vi "Configure Marker.vi"(0 "VISA resource name":refnum<visa-resource-name>, 1 "Marker X Units (0: Seconds)":i32(ring) items=["Seconds", "Hertz"], 2 "Marker Y Position (0.0)":dbl, 5 "Marker Name (1: Marker 1)":i32(ring)=1 items=["Marker 1"=1, "Marker 2"=2], 7 "Marker Type (0: Off)":i32(ring) items=["Off", "Measurement", "Manual", "Waveform", "Binary", "Hex"], 9 "Marker X Position (0.0)":dbl, 11 "error in (no error)":errorcluster, 12 "Marker Source (0: Channel 1)":i32(ring) items=["Channel 1", "Channel 2", "Channel 3", "Channel 4", "Math", "Waveform Memory 1", "Waveform Memory 2"], 13 "Marker Y Units (0: Volts)":i32(ring) items=["Volts", "dB"]) -> (4 "VISA resource name out":refnum<visa-resource-name>, 15 "error out":errorcluster)   [LabVIEW 2010, in "Agilent 2000 3000 X-Series.lvlib"]
doc: "Configures the marker settings."
uses:
  <instrlib>/Agilent 2000 3000 X-Series/Agilent 2000 3000 X-Series.lvlib
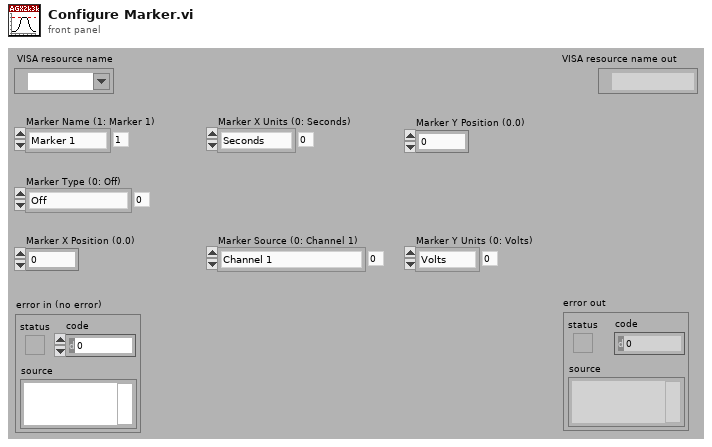
[diagram p1: front panel]
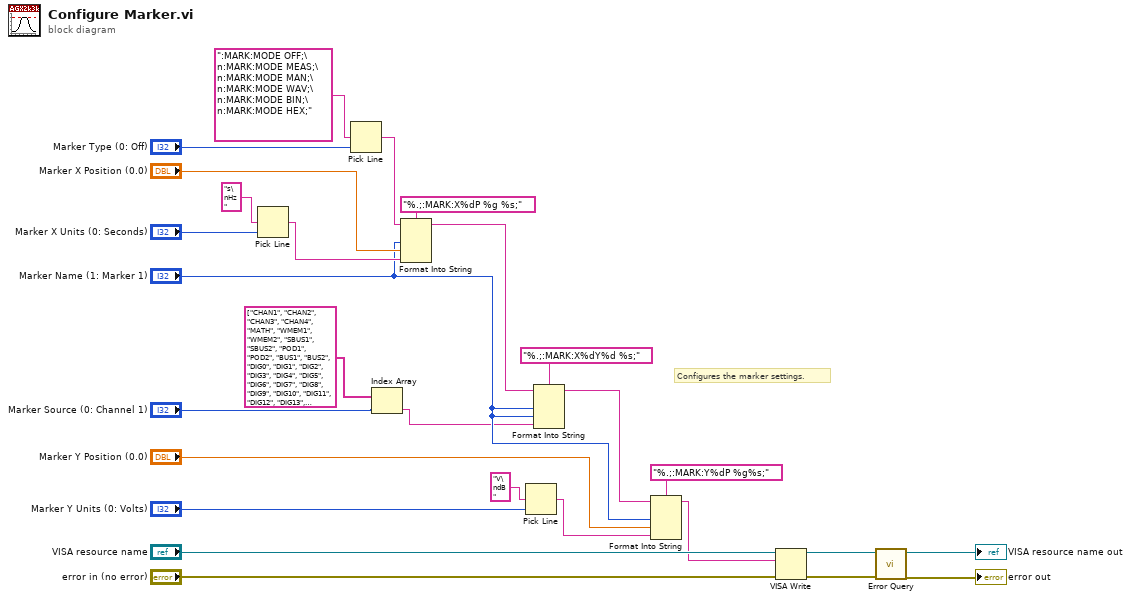
[diagram p0: block diagram]
diagram:
  # "Configures the marker settings."
  n1 = Pick Line(multi-line string="s\nHz", line index="Marker X Units (0: Seconds)") -> (output string=w12:string)  [unwired: 1 out]
  n2 = Pick Line(multi-line string=":MARK:MODE OFF;\n:MARK:MODE MEAS;\n:MARK:MODE MAN;\n:MARK:MODE WAV;\n:MARK:MODE BIN;\n:MARK:MODE HEX;", line index="Marker Type (0: Off)") -> (output string=w23:string)  [unwired: 1 out]
  n3 = Index Array(array=string[] ["CHAN1", "CHAN2", "CHAN3", "CHAN4", "MATH", "WMEM1", "WMEM2", "SBUS1", "SBUS2", "POD1", "POD2", "BUS1", "BUS2", "DIG0", "DIG1", "DIG2", "DIG3", "DIG4", "DIG5", "DIG6", "DIG7", "DIG8", "DIG9", "DIG10", "DIG11", "DIG12", "DIG13", "DIG14", "DIG15", "EXT", "LINE", "WGEN"], index="Marker Source (0: Channel 1)") -> (element=w1:string)
  n4 = Format Into String(format string="%.;:MARK:X%dP %g %s;", initial string=w23, "Marker Name (1: Marker 1)", "Marker X Position (0.0)", w12) -> (resulting string=w11:string)  [unwired: 1 in, 1 out]
  n5 = Pick Line(multi-line string="V\ndB", line index="Marker Y Units (0: Volts)") -> (output string=w8:string)  [unwired: 1 out]
  n6 = Format Into String(format string="%.;:MARK:X%dY%d %s;", initial string=w11, "Marker Name (1: Marker 1)", "Marker Name (1: Marker 1)", w1) -> (resulting string=w6:string)  [unwired: 1 in, 1 out]
  n7 = Format Into String(format string="%.;:MARK:Y%dP %g%s;", initial string=w6, "Marker Name (1: Marker 1)", "Marker Y Position (0.0)", w8) -> (resulting string=w7:string)  [unwired: 1 in, 1 out]
  n8 = VISA Write(VISA resource name="VISA resource name", write buffer=w7, error in (no error)="error in (no error)") -> (VISA resource name out=w16:refnum<visa-resource-name>, error out=w15:errorcluster)  [unwired: 1 out]
  n9 = call <instrlib>:"Error Query.vi"("error in (no error)"=w15, "VISA resource name"=w16) -> ("error out"=→"error out":errorcluster, "VISA resource name out"=→"VISA resource name out":refnum<visa-resource-name>)  [unwired: 8 out]
